vi "EOL CAN_Get_Motor Part Number.vi"(7 "Rx Arbitration Id":u32=402522244 format="%.0x", 8 "error in (no error)":errorcluster, 9 "Tx Arbitration Id":u32=402391172 format="%.0x", 10 "Read Session in":refnum<k21>, 11 "Write Session in":refnum<k21>) -> (0 "error out":errorcluster, 2 "Part Number":string, 4 "Response Good?":bool, 5 "TxRx Data":string[][](array[string]))   [LabVIEW 2018]
uses:
  <vilib>/xnet/xnet.llb/XNET Frame CAN.ctl
  <vilib>/xnet/xnet.llb/XNET Frame Type CAN.ctl
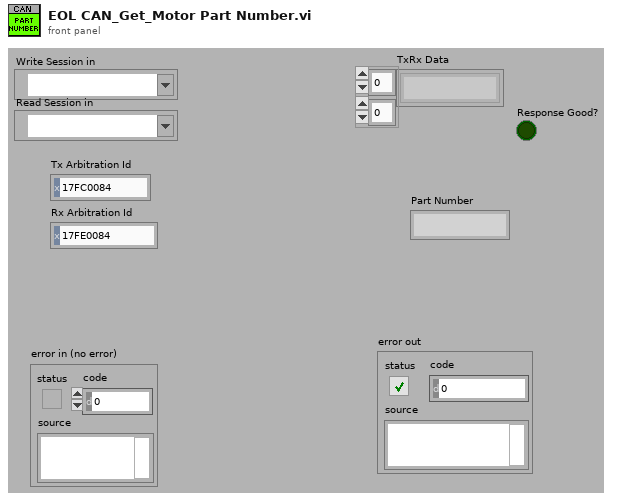
[diagram p1: front panel]
types:
  T1 = typedef "XNET Frame CAN.ctl" = cluster{"timestamp":timestamp, "payload":u8[], "identifier":u32, "type":T2, "extended?":bool, "echo?":bool}
  T2 = typedef "XNET Frame Type CAN.ctl" = u8
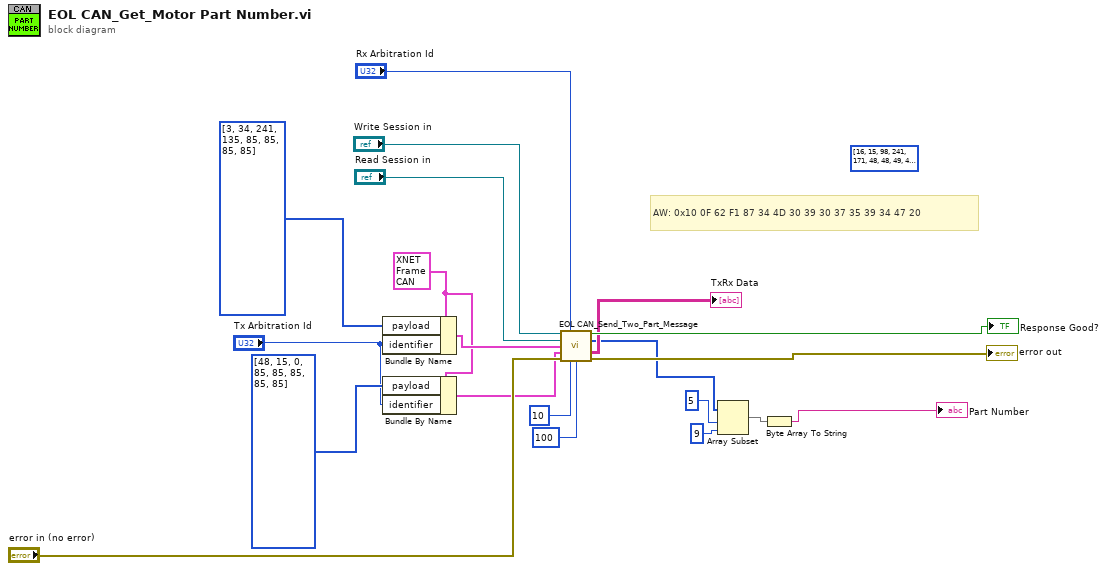
[diagram p0: block diagram]
diagram:
  w8 = T1 {"timestamp"=timestamp(0 s since 1904-01-01), "payload"=[2, 39, 3, 85, 85, 85, 85, 85], "identifier"=402391172, "type"=0, "extended?"=TRUE, "echo?"=FALSE} ("Tx CAN frame 1")
  (unwired) u8[] [16, 15, 98, 241, 171, 48, 48, 49, 48, 48, 48, 48, 53, 48, 48, 48, 51, 170, 170, 170, 170, 170] ("Rx Data")
  # "AW: 0x10 0F 62 F1 87 34 4D 30 39 30 37 35 39 34 47 20"
  n1 = Bundle By Name(cluster=w8, "payload"=u8[] [3, 34, 241, 135, 85, 85, 85, 85] ("Transmit Data"), "identifier"="Tx Arbitration Id") -> (w9:T1)
  n2 = Bundle By Name(cluster=w8, "payload"=u8[] [48, 15, 0, 85, 85, 85, 85, 85] ("Transmit Data"), "identifier"="Tx Arbitration Id") -> (w7:T1)
  n3 = call "EOL CAN_Send_Two_Part_Message.vi"("Write Session in"="Write Session in", "Rx Arbitration Id"="Rx Arbitration Id", "Read Session in"="Read Session in", "Tx CAN frame 1"=w9, "Tx CAN frame 2"=w7, "error in (no error)"="error in (no error)", "Retries"=10, "Msg Wait Time"=u32 100) -> ("Response Good?"=→"Response Good?":bool, "Rx Data"=w14:u8[], "TxRx Data"=→"TxRx Data":string[][], "error out"=→"error out":errorcluster)  [unwired: 4 in]
  n4 = Array Subset(array=w14, index=5, length=9) -> (w2:u8[])
  n5 = Byte Array To String(unsigned byte array=w2) -> (string=→"Part Number":string)
